vi "I32 Image Data to PNG.vi"(8 "error in (no error)":errorcluster, 9 "Image Name Suffix":string="INT Sum", 10 "Image Data":i32[][](array[numeric]), 11 "Reference File Path":path) -> (0 "error out":errorcluster, 2 "Image Out":T1, 3 "PNG File Path":path)   [LabVIEW 2021]
uses:
  <vilib>/vision/Image Controls.llb/IMAQ Image.ctl
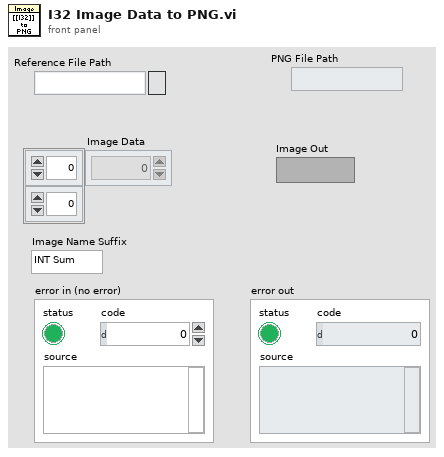
[diagram p1: front panel]
types:
  T1 = typedef "IMAQ Image.ctl" = refnum<image>
  T2 = typedef "Image Type" = u32
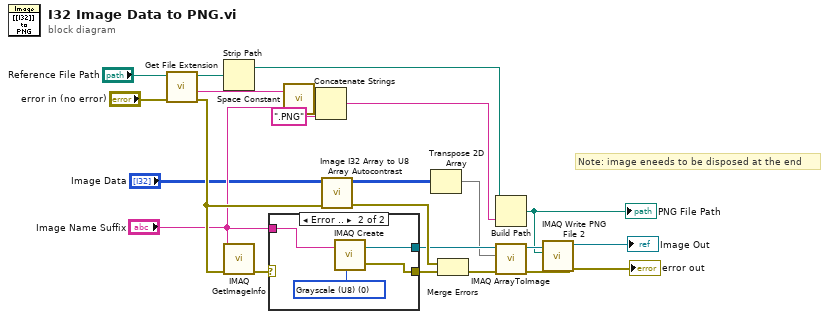
[diagram p0: block diagram]
diagram:
  # "Note: image eneeds to be disposed at the end"
  n1 = call <vilib>:"Get File Extension.vi"("error in (no error)"="error in (no error)", "file"="Reference File Path") -> ("error out"=w20:errorcluster, "filename without extension"=w19:string, "dup file"=w5:path)  [unwired: 5 in, 2 out]
  n2 = Strip Path(path=w5) -> (stripped path=w7:path)  [unwired: 1 out]
  n3 = call "IMAQ GetImageInfo"("error in (no error)"=w20, "Image"="Image Name Suffix") -> ("error out"=w13:errorcluster)  [unwired: 2 in, 7 out]
  n4 = case shown="Error .." w13 {
    selector: w13 -> [w24 _]
    tunnel: [w25 w28] -> w9
    tunnel: [w24 w27] -> w10
    tunnel: "Image Name Suffix" -> [w25 w26]
    frame No Error {
    }
    frame Error {
      w29 = T2 0 items=["Grayscale (U8)", "Grayscale (I16)", "Grayscale (SGL)", "Complex (CSG)", "RGB (U32)", "HSL (U32)", "RGB (U64)", "Grayscale (U16)"] ("Image Type")
      n5 = call "IMAQ Create"("Image Name"=w26, "Image Type"=w29) -> ("New Image"=w28:T1, "error out"=w27:errorcluster)  [unwired: 3 in]
    }
  }
  n6 = call <vilib>:"Space Constant.vi"() -> ("String"=w18:string)
  n7 = Concatenate Strings(w19, w18, "Image Name Suffix", ".PNG" ("string")) -> (w6:string)
  n8 = call "Image I32 Array to U8 Array Autocontrast.vi"("Error In"=w20, "I32 Image"="Image Data") -> ("Error Out"=w23:errorcluster, "U8 5-95% Contrast Enhanced U8 Image"=w21:u8[][])  [unwired: 8 in]
  n9 = Transpose 2D Array(2D array=w21) -> (transposed array=w1:u8[][])
  n10 = Merge Errors(w23, w10) -> (w22:errorcluster)
  n11 = Build Path(base path=w7, name or relative path=w6) -> (appended path=w8:path)
  "PNG File Path" <- w8
  n12 = call "IMAQ ArrayToImage"("error in (no error)"=w22, "Image Pixels (U8)"=w1, "Image"=w9) -> ("error out"=w15:errorcluster, "Image Out"=w12:T1)  [unwired: 7 in]
  n13 = call "IMAQ Write PNG File 2"("error in (no error)"=w15, "File Path"=w8, "Image"=w12) -> ("error out"=→"error out":errorcluster, "Image Out (duplicate)"=→"Image Out":T1)  [unwired: 7 in]
